vi "Scanner Initialize Hardware References.vi"(8 "error in (no error)":errorcluster, 11 "Hardware Resources in":T1={"Link"={"Connection"=enum."USB", "Host or IP address (TCP/IP)"="", "Port (Serial/USB)"="COM1"}, "VISA resource"="", "Writer Queue"=refnum, "Status"=FALSE}) -> (0 "error out":errorcluster, 3 "Hardware Resources out":T1={"Link"={"Connection"=enum."USB", "Host or IP address (TCP/IP)"="", "Port (Serial/USB)"="COM1"}, "VISA resource"="", "Writer Queue"=refnum, "Status"=FALSE})   [LabVIEW 2020, in "Hiden Scanner.lvlib"]
doc: "Initialize the hardware references."
uses:
  Hiden Scanner.lvlib
  Scanner Hardware Configuration.ctl
  support/Message Queue/Message Cluster.ctl
  <instrlib>/Hiden/Hiden MS.lvlib
  support/Message Queue/Message Queue.lvlib
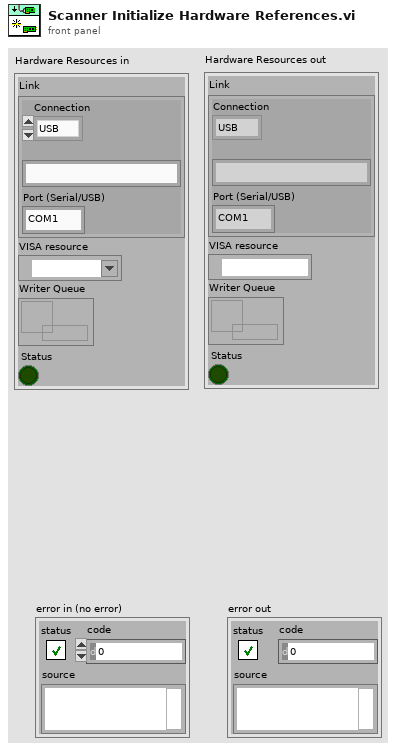
[diagram p1: front panel]
types:
  T1 = typedef "Hiden Scanner.lvlib/Scanner Hardware Configuration.ctl" = cluster{"Link":cluster{"Connection":enum16{"Serial", "TCP/IP", "USB"}, "Host or IP address (TCP/IP)":string, "Port (Serial/USB)":string}, "VISA resource":refnum<visa-resource-name>, "Writer Queue":refnum<queue>, "Status":bool}
  T2 = cluster{"Connection":enum16{"Serial", "TCP/IP", "USB"}, "Host or IP address (TCP/IP)":string, "Port (Serial/USB)":string}
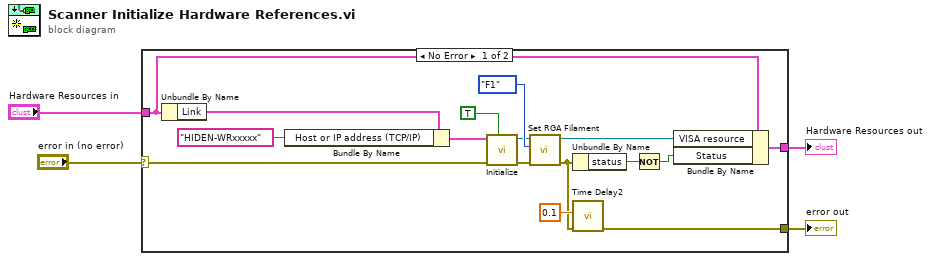
[diagram p0: block diagram]
diagram:
  n1 = case shown="No Error" "error in (no error)" {
    selector: "error in (no error)" -> [w12 w21]
    tunnel: [w16 w21] -> w3
    tunnel: "Hardware Resources in" -> [w19 w22]
    tunnel: [w20 w22] -> w1
    frame No Error {
      n2 = Unbundle By Name(w19) -> ("Link"=w13:T2)
      n3 = Bundle By Name(cluster=w13, "Host or IP address (TCP/IP)"="HIDEN-WRxxxxx") -> (w11:T2)
      n4 = call <instrlib>:"Initialize.vi"("Enable comms logging (F)"=TRUE, "error in (no error)"=w12, "Link"=w11) -> ("error out"=w6:errorcluster, "Connection"=w8:refnum<visa-resource-name>)  [unwired: 7 in]
      n5 = call <instrlib>:"Set RGA Filament.vi"("error in (no error)"=w6, "Filament"=enum16{"F1", "F2"}."F1", "Connection"=w8) -> ("error out"=w5:errorcluster, "Connection (dup)"=w7:refnum<visa-resource-name>)  [unwired: 7 in]
      n6 = Unbundle By Name(w5) -> ("status"=w17:bool)
      n7 = call "Time Delay2"("error in (no error)"=w5, "Delay Time (s)"=0.1) -> ("error out"=w16:errorcluster)  [unwired: 9 in]
      n8 = Not(x=w17) -> (.not. x?=w18:bool)
      n9 = Bundle By Name(cluster=w19, "VISA resource"=w7, "Status"=w18) -> (w20:T1)
    }
    frame Error {
    }
  }
  "Hardware Resources out" <- w1
  "error out" <- w3
